vi "Init.vi"(8 "error in (no error)":errorcluster, 11 "uService Template in":refnum<class "Simple Device Manager.lvclass">) -> (0 "error out":errorcluster, 3 "uService Template out":refnum<class "Simple Device Manager.lvclass">)   [LabVIEW 2020, in "Simple Device Manager.lvlib" / "Simple Device Manager.lvclass"]
uses:
  Simple Device Manager.lvclass
  Consumer Case Selector.ctl
  TALOS/TALOS_PPL.lvlibp/Ancestor/Ancestor/Infinite Message Selector.ctl
  Simple Device Manager.lvclass/Simple Device Manager.ctl
  TALOS/TALOS_PPL.lvlibp/Father of all uServices/Father of all uServices/Father of all uServices.lvclass
  Hardware/Simple Device/Simple Device.lvclass
  TALOS/TALOS_PPL.lvlibp
  TALOS/TALOS_PPL.lvlibp/Ancestor/Ancestor/Ancestor.lvclass
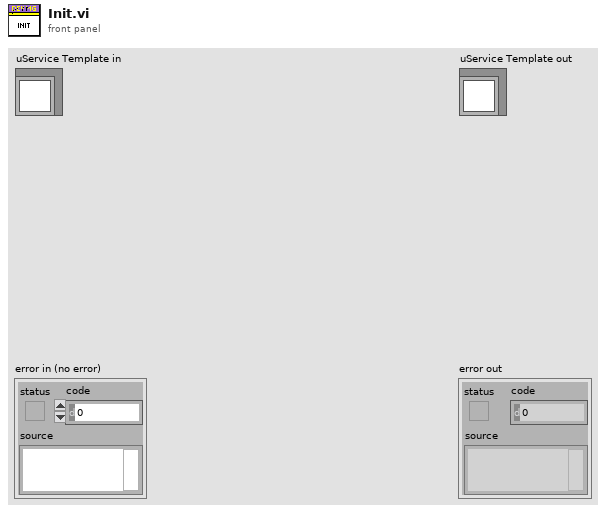
[diagram p1: front panel]
types:
  T1 = typedef "TALOS_PPL.lvlibp/Ancestor.lvlib/Ancestor.lvclass/Infinite Message Selector.ctl" = enum16{"Start", "Stop", "Check", "Flush (Stop all)", "Init"}
  T2 = typedef "Simple Device Manager.lvlib/Simple Device Manager.lvclass/Consumer Case Selector.ctl" = enum16{"Set current", "Check status", "Check temperature"}
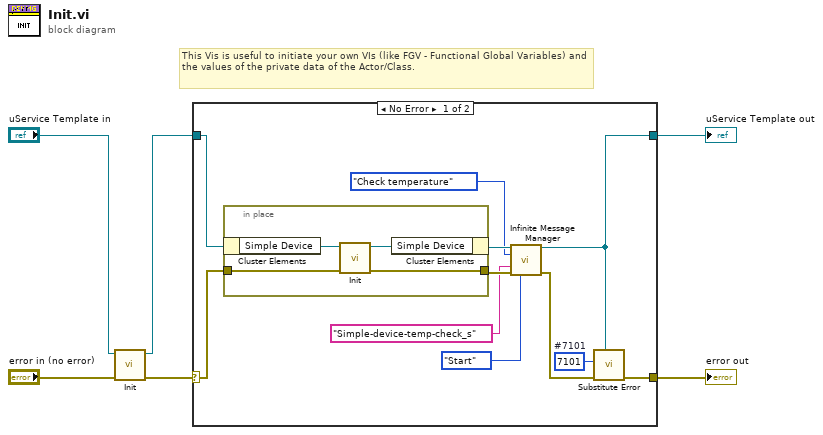
[diagram p0: block diagram]
diagram:
  # "This Vis is useful to initiate your own VIs (like FGV - Functional Global Variables) and the values of the private data of the Actor/Class."
  n1 = call-parent "Init.vi"("error in (no error)"="error in (no error)", "uService Template in"="uService Template in") -> ("error out"=w3:errorcluster, "uService Template out"=w1:refnum<class "Simple Device Manager.lvclass">)  [unwired: 8 in]
  n2 = case shown="No Error" w3 {
    selector: w3 -> [w16 w22]
    tunnel: w1 -> [w17 w23]
    tunnel: [w13 w23] -> w6
    tunnel: [w15 w22] -> w5
    frame No Error {
      w7 = 7101  # #7101
      n3 = in-place {
        in-place-border: w16 -> [w19]
        in-place-border: [w18] -> w11
        n4 = in-place-cluster #1(w17) -> ("Simple Device"=w21:refnum<class "Simple Device.lvclass">)
        n5 = call-dynamic "Init.vi"("error in (no error)"=w19, "Simple Device in"=w21) -> ("error out"=w18:errorcluster, "Simple Device out"=w20:refnum<class "Simple Device.lvclass">)  [unwired: 8 in]
        n6 = in-place-cluster #1("Simple Device"=w20) -> (w14:refnum<class "Simple Device Manager.lvclass">)
      }
      n7 = call-dynamic "Infinite Message Manager.vi"("Father of all uServices in"=w14, "Consumer Case Selector"=Consumer_Case_Selector."Check temperature", "Tau parameter"="Simple-device-temp-check_s", "error in (no error)"=w11, "Infinite Message Selector"=Infinite_Message_Selector."Start") -> ("Father of all uServices out"=w13:refnum<class "Simple Device Manager.lvclass">, "error out"=w12:errorcluster)  [unwired: 8 in, 1 out]
      n8 = call "Substitute Error.vi"("LabVIEW Object"=w13, "error in (no error)"=w12, "Error Code"=w7) -> ("error out"=w15:errorcluster)  [unwired: 8 in]
    }
    frame Error {
    }
  }
  "error out" <- w5
  "uService Template out" <- w6
